vi "ReadTXTSubViI.vi"() -> ()   [LabVIEW 2023]
uses:
  <vilib>/Utility/file.llb/Read Delimited Spreadsheet (string).vi
panel:
  out "output cluster 2":T1
  out "x = y? 2":T2
  in  "Haslo 2":string
  in  "Login":string
  out "x = y?":T3
  out "output cluster":T4
  out "subarray":string[][](array[string])
  in  "delimiter (\\t)":string="\t"
  in  "format (%s)":string="%s"
  out "all rows":string[][](array[string])
  in  "Path":path
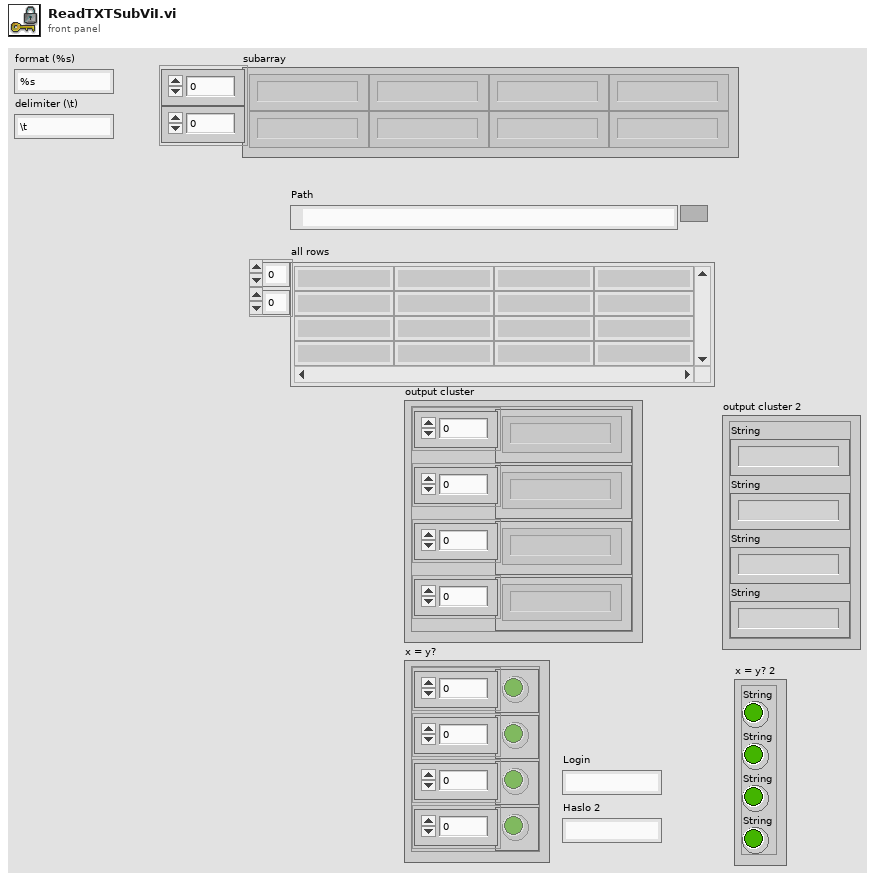
[diagram p1: front panel]
types:
  T1 = cluster{"String":string, "String":string, "String":string, "String":string}
  T2 = cluster{"String":bool, "String":bool, "String":bool, "String":bool}
  T3 = cluster{"Array":bool[], "Array":bool[], "Array":bool[], "Array":bool[]}
  T4 = cluster{"Array":string[], "Array":string[], "Array":string[], "Array":string[]}
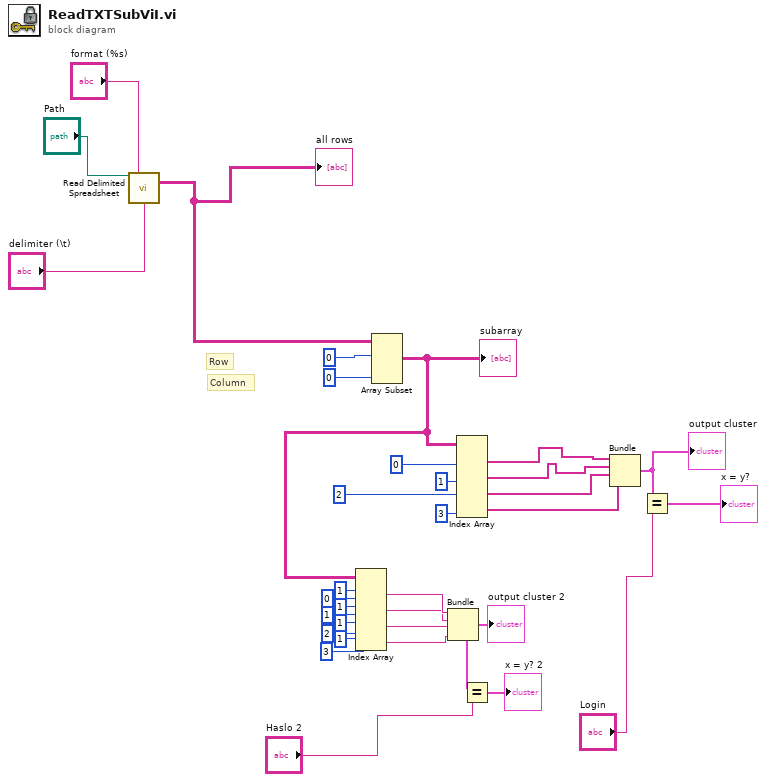
[diagram p0: block diagram]
diagram:
  # "Column"
  # "Row"
  n1 = call-poly <vilib>:"Read Delimited Spreadsheet.vi"("file path (dialog if empty)"="Path", "format (%s)"="format (%s)", "delimiter (\\t)"="delimiter (\\t)") -> ("all rows"=w30:string[][])  [unwired: 7 in, 5 out]
  "all rows" <- w30
  n2 = Array Subset(array=w30, index (row)=0 ("index"), index (col)=0 ("index")) -> (w16:string[][])  [unwired: 2 in]
  "subarray" <- w16
  n3 = Index Array(array=w16, index (row) #1=1 ("index (row)"), index (col) #1=0 ("disabled index (col)"), index (row) #2=1 ("index (row)"), index (col) #2=1 ("disabled index (col)"), index (row) #3=1 ("index (row)"), index (col) #3=2 ("disabled index (col)"), index (row) #4=1 ("index (row)"), index (col) #4=3 ("disabled index (col)")) -> (element #1=w14:string, element #2=w13:string, element #3=w12:string, element #4=w11:string)
  n4 = Bundle("String"=w14, "String"=w13, "String"=w12, "String"=w11) -> (w10:T1)  [unwired: 1 in]
  "output cluster 2" <- w10
  n5 = Index Array(array=w16, index (col) #1=0 ("disabled index (col)"), index (col) #2=1 ("disabled index (col)"), index (col) #3=2 ("disabled index (col)"), index (col) #4=3 ("index (col)")) -> (element #1=w27:string[], element #2=w25:string[], element #3=w24:string[], element #4=w23:string[])  [unwired: 4 in]
  n6 = Equal?(x=w10, y="Haslo 2") -> (x = y?=→"x = y? 2":T2)
  n7 = Bundle(w27, w25, w24, w23) -> (w26:cluster{string[], string[], string[], string[]})  [unwired: 1 in]
  "output cluster" <- w26
  n8 = Equal?(x=w26, y="Login") -> (x = y?=→"x = y?":cluster{bool[], bool[], bool[], bool[]})
